vi "Magnet pulse mode test.vi"() -> ()   [LabVIEW 2021]
panel:
  in  "stop":bool
  in  "Off Delay Time (s)":dbl=1.0 caption="Delay Time (s)"
  out "error out":errorcluster
  in  "On Time (s)":dbl=1.0 caption="Delay Time (s)"
  in  "Field Rate mT per sec":dbl=0.1 format="%#_13g"
  in  "Field Target mT":dbl format="%#_13g"
  in  "Magnet Device Select":string(combo)="Elsa Magnet"
  in  "error in (no error)":errorcluster
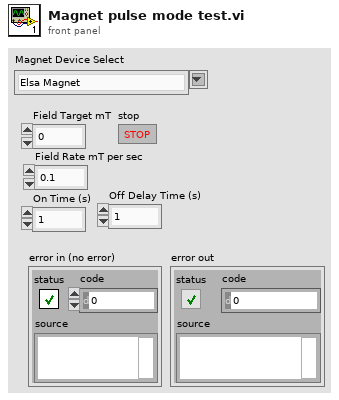
[diagram p1: front panel]
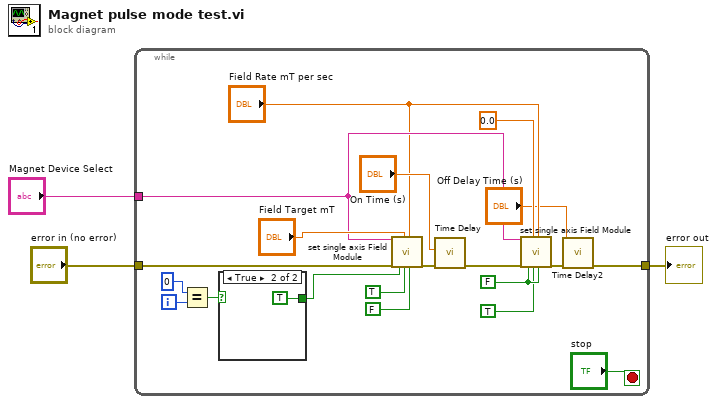
[diagram p0: block diagram]
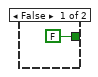
[diagram p2: hidden frame]
diagram:
  n1 = while {
    tunnel: "error in (no error)" -> [w21]
    tunnel: "Magnet Device Select" -> [w12]
    tunnel: [w6] -> w1
    i -> [w23]
    stop <- "stop" stop-if-true
    w9 = FALSE ("Init")
    n2 = Equal?(x=0, y=w23) -> (x = y?=w22:bool)
    n3 = case shown="True" w22 {
      tunnel: [FALSE ("Init") TRUE ("Init")] -> w19
      frame False {
      }
      frame True {
      }
    }
    n4 = call "set single axis Field Module.vi"("Field Device Select"=w12, "error in (no error)"=w21, "Init"=w19, "Field Target mT or dBm"="Field Target mT", "Exec"=TRUE, "Field Rate mT per sec"="Field Rate mT per sec", "final"=FALSE) -> ("error out"=w15:errorcluster)  [unwired: 12 in]
    n5 = call "Time Delay"("error in (no error)"=w15, "Delay Time (s)"="On Time (s)") -> ("error out"=w13:errorcluster)  [unwired: 9 in]
    n6 = call "set single axis Field Module.vi"("Field Device Select"=w12, "error in (no error)"=w13, "Init"=w9, "Field Target mT or dBm"=0.0 ("Field Target mT"), "Exec"=TRUE, "Field Rate mT per sec"="Field Rate mT per sec", "final"=w9) -> ("error out"=w7:errorcluster)  [unwired: 12 in]
    n7 = call "Time Delay2"("error in (no error)"=w7, "Delay Time (s)"="Off Delay Time (s)") -> ("error out"=w6:errorcluster)  [unwired: 9 in]
  }
  "error out" <- w1
